vi "arduinoOpenComPort.vi"(8 "Error In":errorcluster, 10 "Baud Rate":u32=9600, 11 "COM Port":refnum<visa-resource-name>="COM4") -> (0 "error out":errorcluster, 3 "VISA resource name out":refnum<visa-resource-name>)   [LabVIEW 2019]
uses:
  <vilib>/Instr/_visa.llb/VISA Configure Serial Port (Instr).vi
panel:
  out "Port Available?":bool
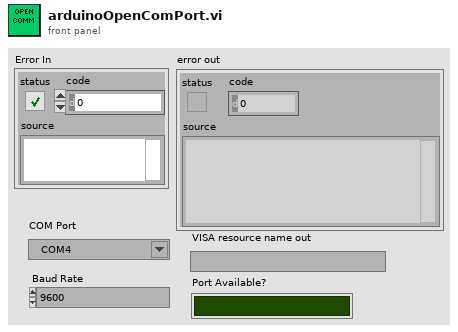
[diagram p1: front panel]
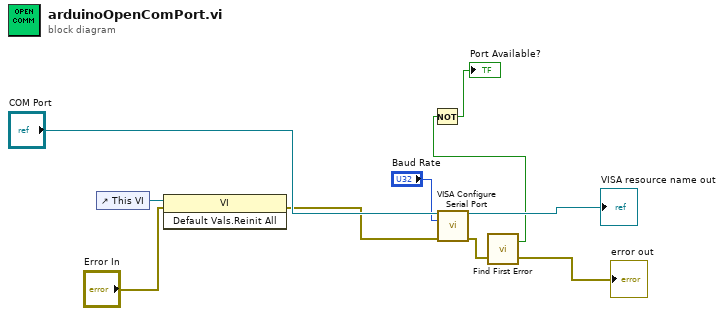
[diagram p0: block diagram]
diagram:
  n1 = control-ref of="This VI"() -> (w10:refnum<vi>)
  n2 = invoke class="VI" method="Default Vals.Reinit All"(reference=w10, error in="Error In") -> (error out=w7:errorcluster)  [unwired: 1 in, 2 out]
  n3 = call-poly "VISA Configure Serial Port"("VISA resource name"="COM Port", "baud rate (9600)"="Baud Rate", "error in (no error)"=w7) -> ("VISA resource name out"=→"VISA resource name out":refnum<visa-resource-name>, "error out"=w5:errorcluster)  [unwired: 11 in]
  n4 = call <vilib>:"Find First Error.vi"("error in (no error)"=w5) -> ("error out"=→"error out":errorcluster, "error?"=w4:bool)  [unwired: 3 in]
  n5 = Not(x=w4) -> (.not. x?=→"Port Available?":bool)
